vi "gui for running status.vi"() -> ()   [LabVIEW 2022 SP3]
uses:
  counterweight load control.ctl
  status bar control.ctl
panel:
  out "Slide 6":u8(slide)=100 scale=0.0..100.0
  out "Slide 5":u8(slide)=100 scale=0.0..100.0
  out "Slide 4":u8(slide)=53 scale=0.0..100.0
  in  "Stop Button 2":bool
  out "Numeric 4":dbl format="%d%"
  in  "Gauge 4":dbl(knob)=1.2869315802184793e-48 scale=0.0..100.0
  in  "Stop Button":bool
  out "Numeric 3":dbl format="%d%"
  in  "Gauge 3":T1=1.2869315802184793e-48 scale=0.0..100.0
  out "?":T2 scale=0.0..6.0
  out "?":string
  in  "Close Button":bool
  out "?":picture
  out "?":picture
  in  "Table 2":string[][](table)
  # "0"
  # "Auto Running Mode"
  # "Running Cycle"
  # "Overall Cycle Bar"
  # "100"
  # "0"
  # "X axis"
  # "Y axis"
  # "X axis progress"
  # "Y axis progress"
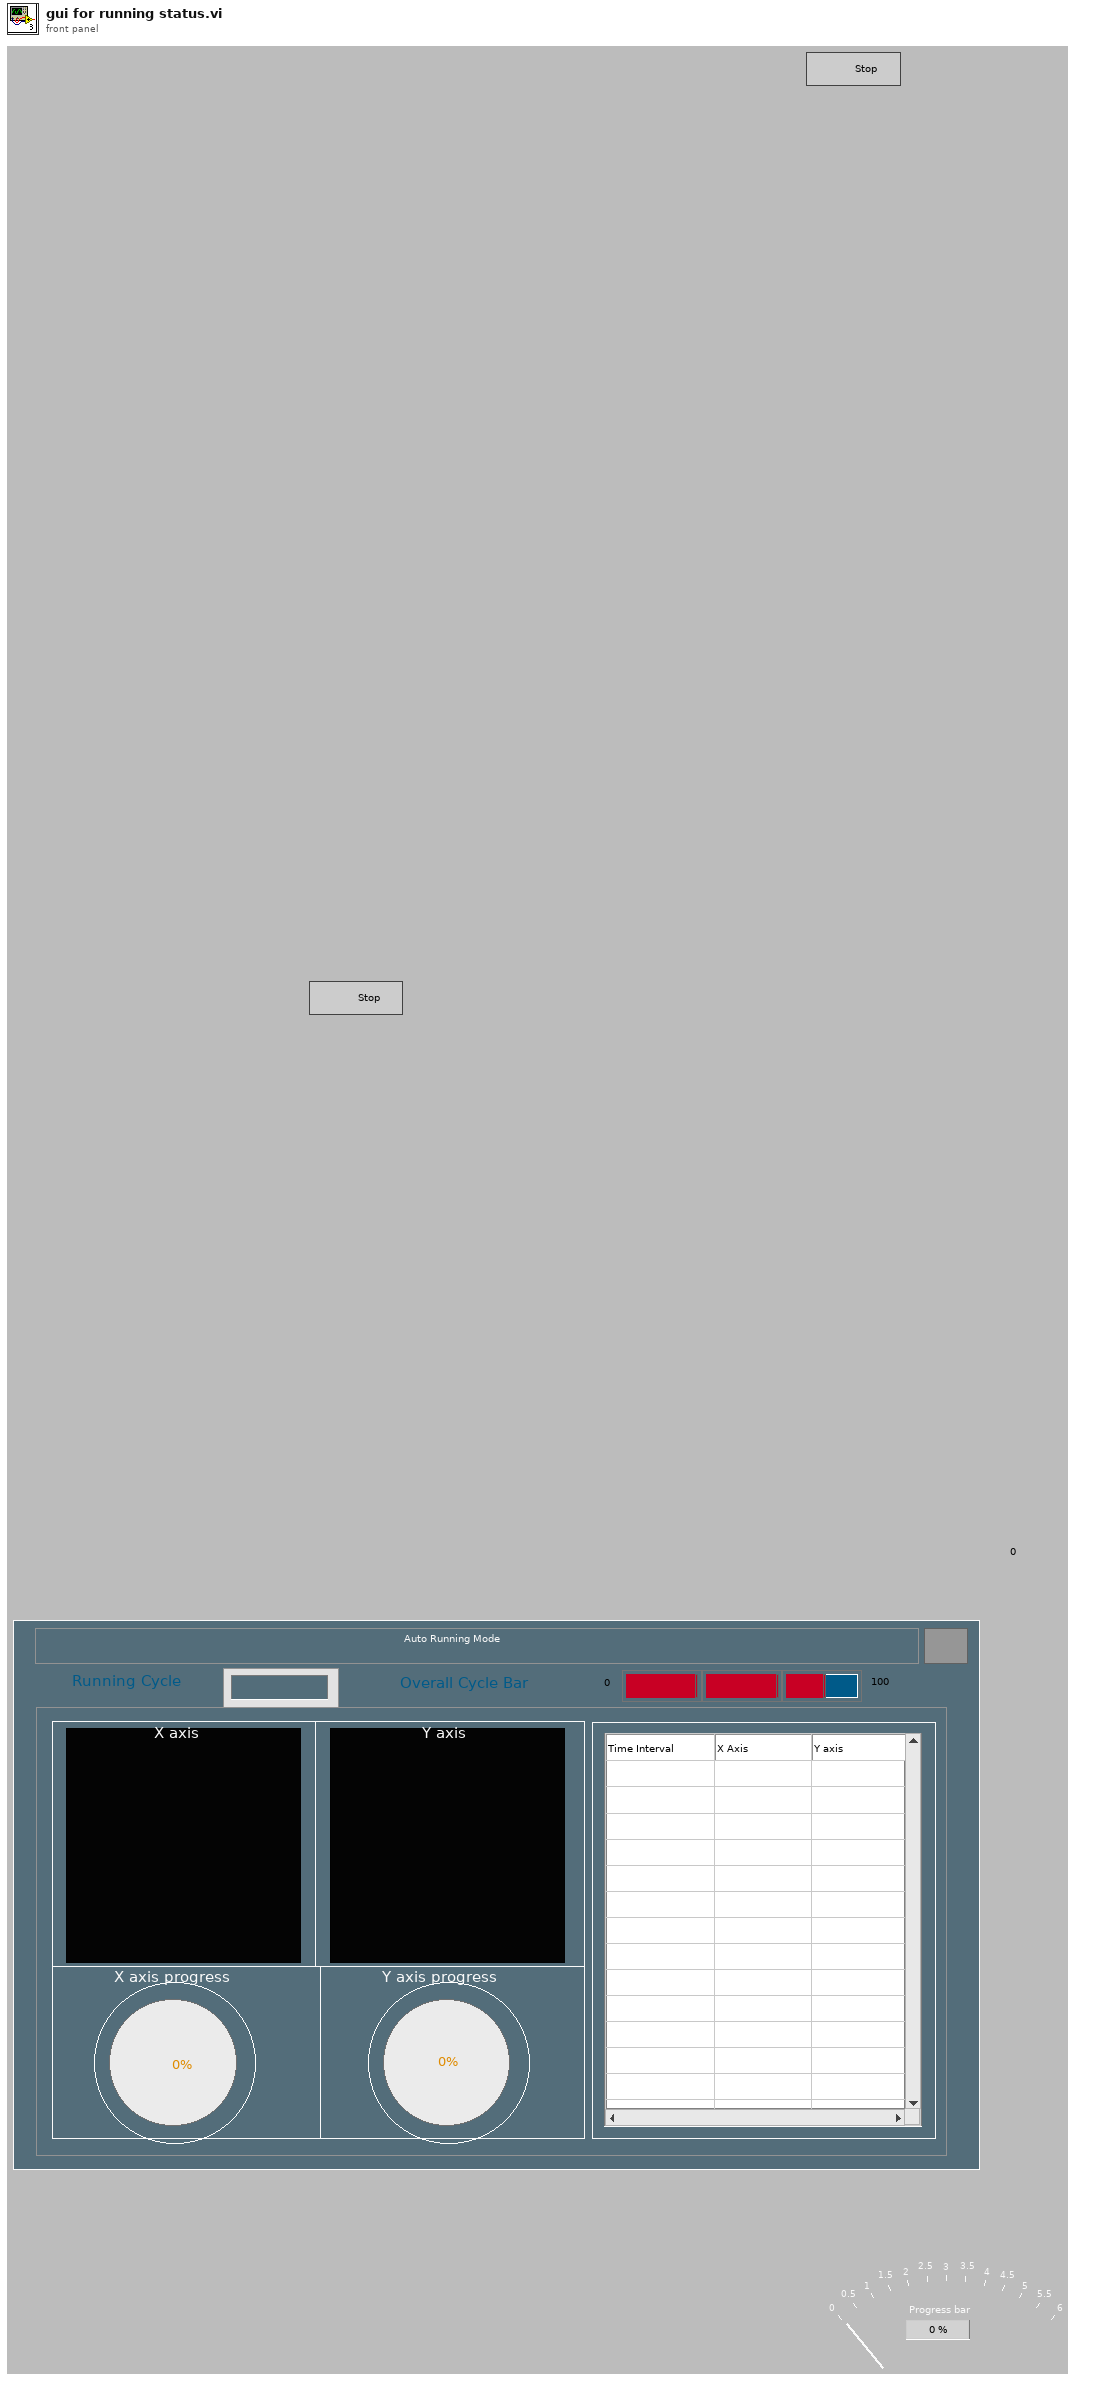
[diagram p1: front panel]
types:
  T1 = typedef "status bar control.ctl" = dbl
  T2 = typedef "counterweight load control.ctl" = dbl
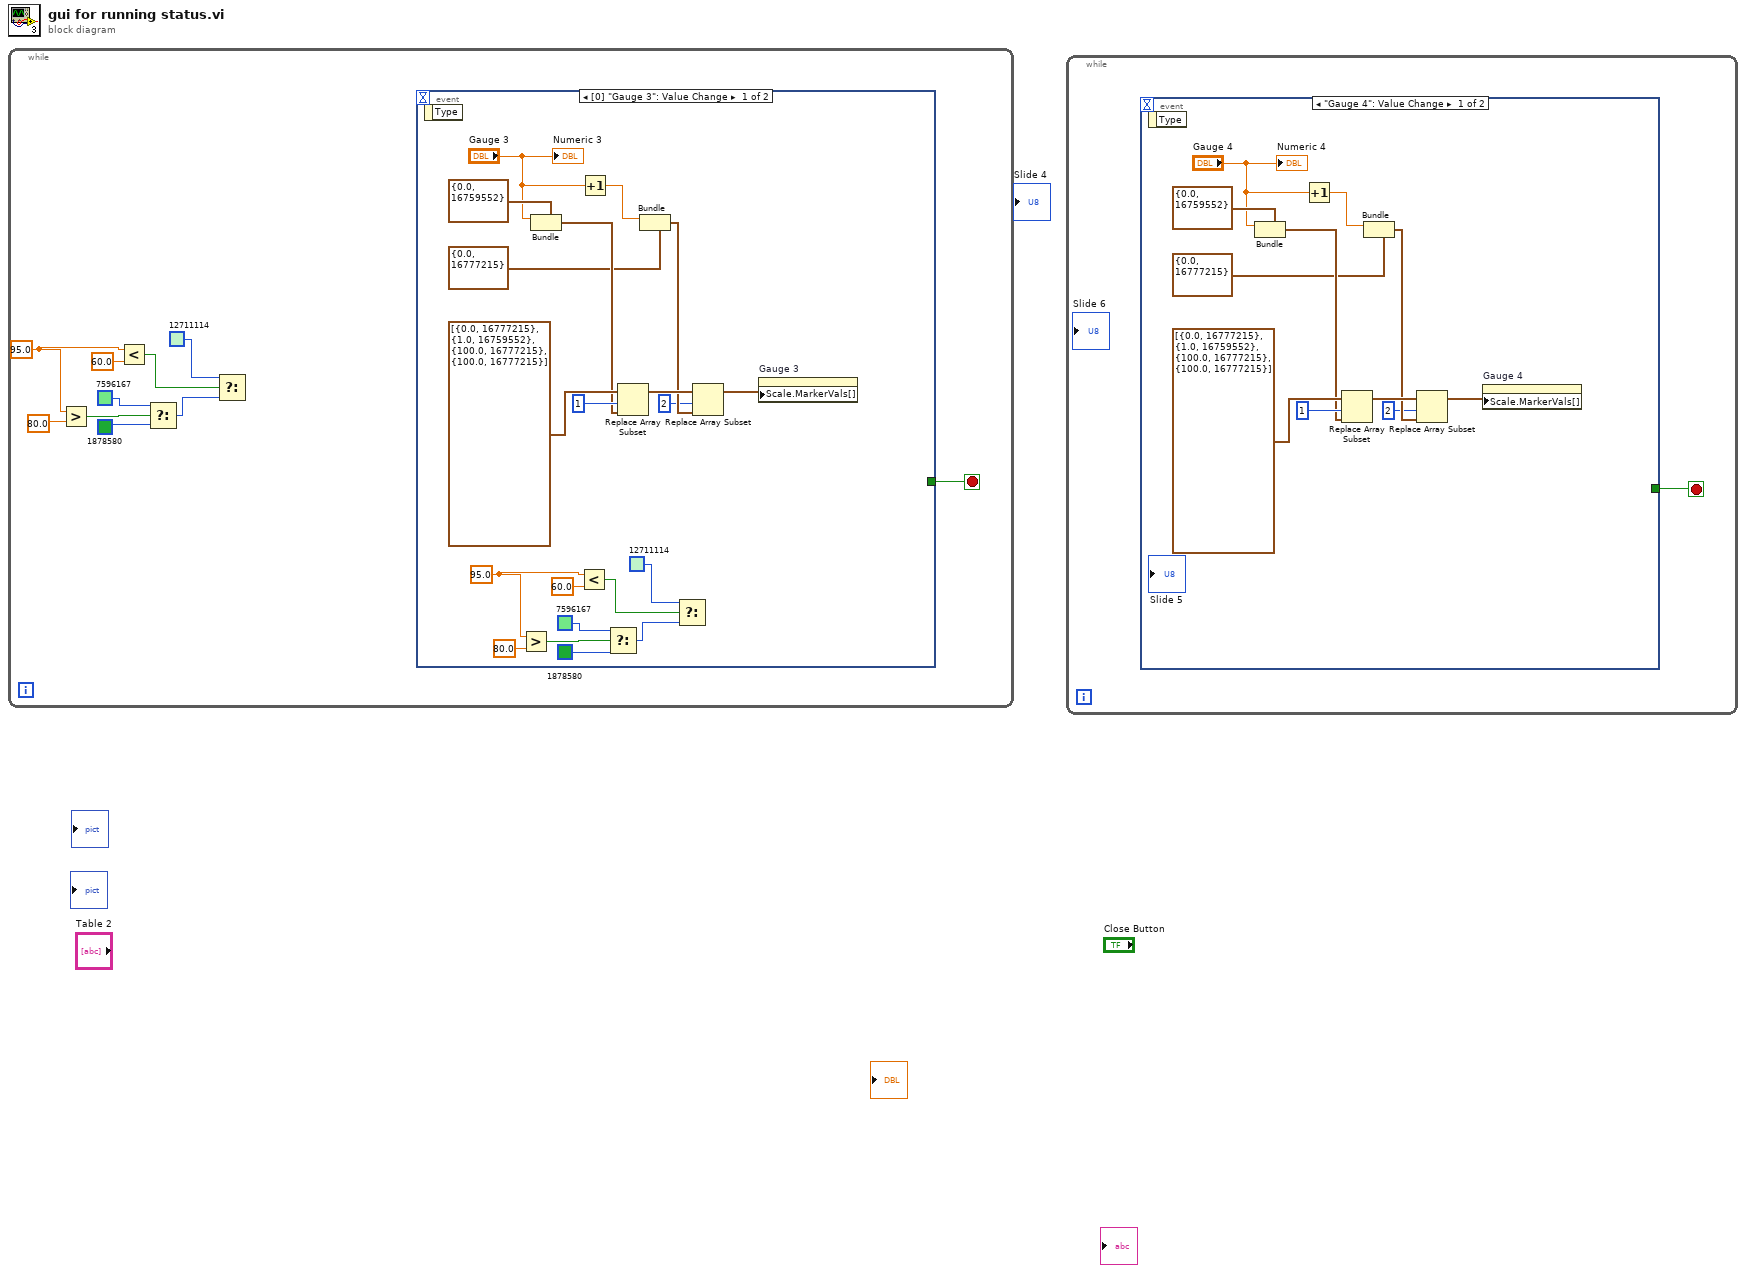
[diagram p0: block diagram]
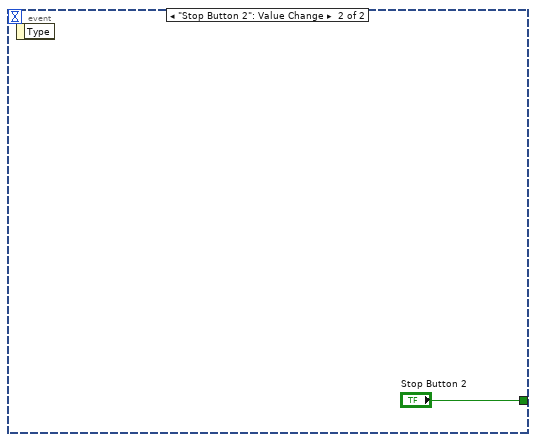
[diagram p2: hidden frame]
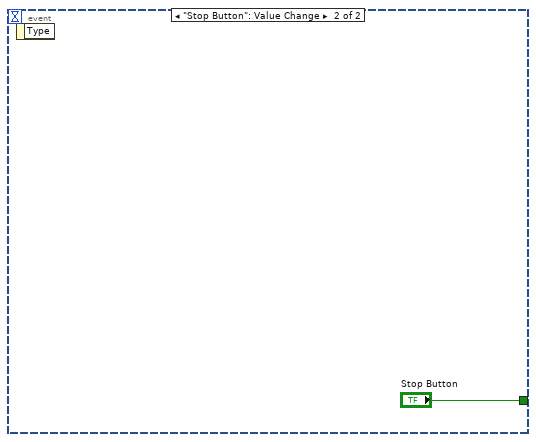
[diagram p3: hidden frame]
diagram:
  n1 = while {
    stop <- w10 stop-if-true
    w7 = 95.0 ("Numeric")
    n2 = Greater?(x=w7, y=80.0) -> (0:w4:bool)
    n3 = Less?(x=w7, y=60.0) -> (x < y?=w5:bool)
    n4 = Select(t=u32 7596167, s=w4, f=u32 1878580) -> (s? t:f=w3:u32)
    n5 = Select(t=u32 12711114, s=w5, f=w3) -> ()  [unwired: 1 out]
    n6 = event shown="[0] \"Gauge 3\": Value Change" {
      selector: _ -> [_ _]
      dyn-events: _ -> [_ _]
      timeout: _ -> [_ _]
      tunnel: [_ "Stop Button"] -> w10
      event Value Change {
        w13 = 95.0 ("Numeric")
        n7 = event-data() -> ()  [unwired: 1 in, 1 out]
        n8 = Greater?(x=w13, y=80.0) -> (0:w18:bool)
        n9 = Bundle(cluster=cluster{dbl, i32} {0.0, 16759552}, "Gauge 3") -> (w28:cluster{dbl, i32})  [unwired: 1 in]
        n10 = Less?(x=w13, y=60.0) -> (x < y?=w17:bool)
        n11 = Increment(x="Gauge 3") -> (x+1=w26:T1)
        n12 = Select(t=u32 7596167, s=w18, f=u32 1878580) -> (s? t:f=w19:u32)
        n13 = Replace Array Subset(array=cluster{dbl, u32}[] [{0.0, 16777215}, {1.0, 16759552}, {100.0, 16777215}, {100.0, 16777215}] ("Scale.Marker Values[]"), new element=w28, index=1) -> (w24:cluster{dbl, u32}[])
        n14 = Bundle(cluster=cluster{dbl, i32} {0.0, 16777215}, w26) -> (w23:cluster{dbl, i32})  [unwired: 1 in]
        n15 = Select(t=u32 12711114, s=w17, f=w19) -> ()  [unwired: 1 out]
        n16 = Replace Array Subset(array=w24, new element=w23, index=2) -> (w21:cluster{dbl, u32}[])
        n17 = property on="Gauge 3" class="Knob (strict)"("Scale.MarkerVals[]"=w21) -> ()  [unwired: 2 in, 2 out]
        "Numeric 3" <- "Gauge 3"
      }
      event "Stop Button": Value Change {
        n18 = event-data() -> ()  [unwired: 1 in, 1 out]
      }
    }
  }
  n19 = while {
    stop <- w32 stop-if-true
    n20 = event shown="[0] \"Gauge 4\": Value Change" {
      selector: _ -> [_ _]
      dyn-events: _ -> [_ _]
      timeout: _ -> [_ _]
      tunnel: [_ "Stop Button 2"] -> w32
      event "Gauge 4": Value Change {
        n21 = event-data() -> ()  [unwired: 1 in, 1 out]
        n22 = Bundle(cluster=cluster{dbl, i32} {0.0, 16759552}, "Gauge 4") -> (w41:cluster{dbl, i32})  [unwired: 1 in]
        n23 = Increment(x="Gauge 4") -> (x+1=w39:dbl)
        n24 = Replace Array Subset(array=cluster{dbl, u32}[] [{0.0, 16777215}, {1.0, 16759552}, {100.0, 16777215}, {100.0, 16777215}] ("Scale.Marker Values[]"), new element=w41, index=1) -> (w37:cluster{dbl, u32}[])
        n25 = Bundle(cluster=cluster{dbl, i32} {0.0, 16777215}, w39) -> (w36:cluster{dbl, i32})  [unwired: 1 in]
        n26 = Replace Array Subset(array=w37, new element=w36, index=2) -> (w34:cluster{dbl, u32}[])
        n27 = property on="Gauge 4" class="Knob (strict)"("Scale.MarkerVals[]"=w34) -> ()  [unwired: 2 in, 2 out]
        "Numeric 4" <- "Gauge 4"
      }
      event "Stop Button 2": Value Change {
        n28 = event-data() -> ()  [unwired: 1 in, 1 out]
      }
    }
  }
